vi "Write Move Motor.vi"(8 "error in (no error)":errorcluster, 9 "Desired Value":variant, 10 "Motor":T1, 11 "AISAS Mech in":refnum<class "AISAS Mech.lvclass">) -> (0 "error out":errorcluster, 3 "AISAS Mech out":refnum<class "AISAS Mech.lvclass">)   [LabVIEW 2014, in "AISAS Mech.lvclass"]
uses:
  AISAS Mech.lvclass
  Controls/motor.ctl
  AISAS Mech.lvclass/AISAS Mech.ctl
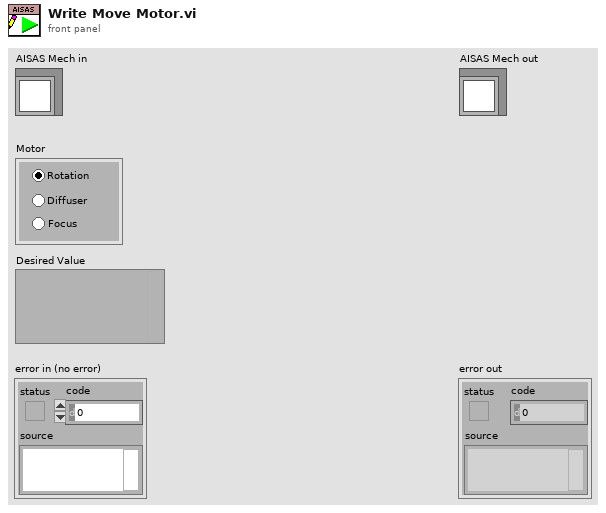
[diagram p1: front panel]
types:
  T1 = typedef "motor.ctl" = enum32{"Rotation", "Diffuser ", "Focus"}
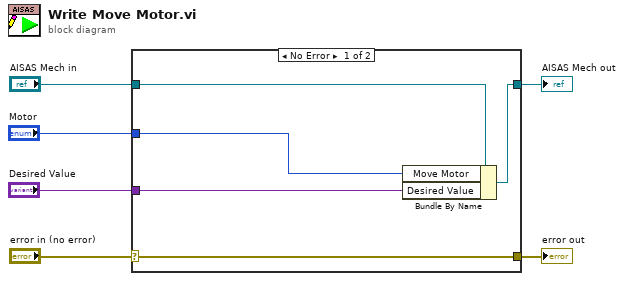
[diagram p0: block diagram]
diagram:
  n1 = case shown="No Error" "error in (no error)" {
    selector: "error in (no error)" -> [w11 w12]
    tunnel: [w11 w12] -> w5
    tunnel: [w9 w13] -> w3
    tunnel: "AISAS Mech in" -> [w10 w13]
    tunnel: "Motor" -> [w8 _]
    tunnel: "Desired Value" -> [w7 _]
    frame No Error {
      n2 = Bundle By Name(cluster=w10, "Move Motor"=w8, "Desired Value"=w7) -> (w9:refnum<class "AISAS Mech.lvclass">)
    }
    frame Error {
    }
  }
  "error out" <- w5
  "AISAS Mech out" <- w3
